vi "AlliGator Phasor Plot Multiplication Window.vi"(8 "Error In":errorcluster, 11 "Phasor Graph":refnum<vi>) -> (0 "Error Out":errorcluster, 1 "Cancelled":bool, 2 "Phasor Plot Destination Output":T1, 3 "Phasor Plot Algebra Output":T2 {"1-Exp Lifetime" min=0.0; "Delay" min=0.0})   [LabVIEW 2021, in "AlliGator Phasor Graph.lvlib"]
doc: "UI to let the user define algebraic operations to apply to Phasor Plots in the Phasor Graph."
uses:
  AlliGator Phasor Graph.lvlib
  AlliGator 2-Phasor Plot Multiplication.ctl
  Phasor/Phasor Operation.ctl
  Phasor/Phasor (g, s).ctl
  Phasor/Phasor (m, phi).ctl
  Phasor/Phasor Representation.ctl
  AlliGator Phasor Plot Destination.ctl
  Graphs/XY Graph/XY Graph Add-Ons.lvlib
  Phasor/Phasor.lvlib
panel:
  in  "Phasor Plot Destination":T1
  in  "Phasor Plot Algebra":T2 {"1-Exp Lifetime" min=0.0; "Delay" min=0.0; "Phasor Plot 2" items=["", "Phasor 1", "Phasor 2"]; "Phasor Plot 1" items=["", "Phasor 1", "Phasor 2"]}
  in  "OK":bool
  in  "Cancel":bool
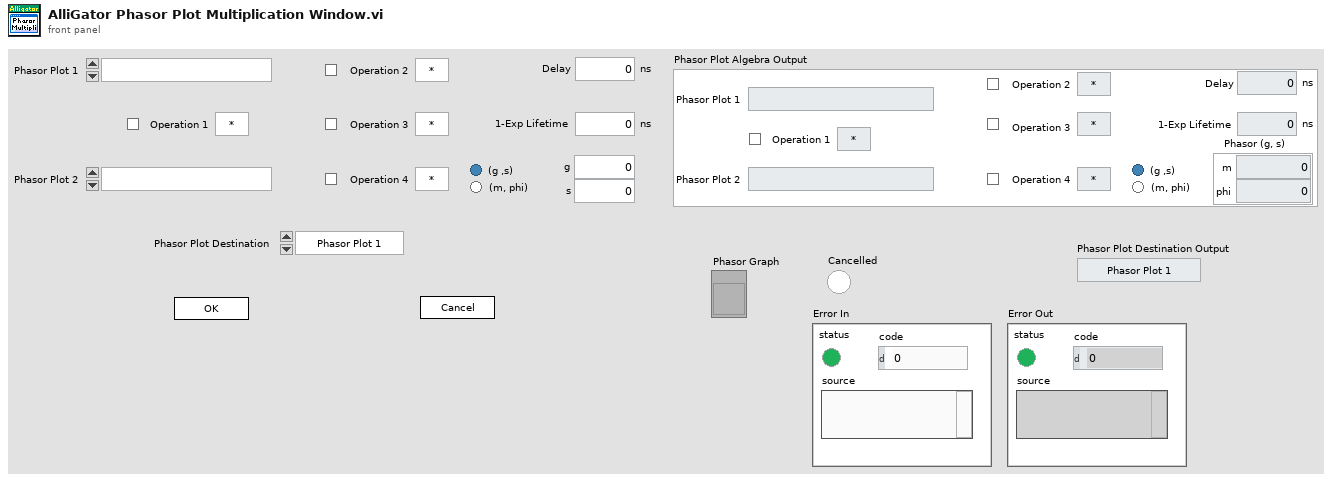
[diagram p1: front panel]
types:
  T1 = typedef "AlliGator Phasor Graph.lvlib/AlliGator Phasor Plot Destination.ctl" = enum32{"Phasor Plot 1", "Phasor Plot 2", "New Phasor Plot"}
  T2 = typedef "AlliGator Phasor Graph.lvlib/AlliGator 2-Phasor Plot Multiplication.ctl" = cluster{"Phasor Plot 1":u16, "Operation 1":T3, "Phasor Plot 2":u16, "Operation 2":T3, "Delay":dbl[unit], "Operation 3":T3, "1-Exp Lifetime":dbl[unit], "Operation 4":T3, "Phasor (g, s)":T4, "Phasor (m, phi)":T5, "Phasor Representation":T6, "Use Operation 1":bool, "Use Operation 2":bool, "Use Operation 3":bool, "Use Operation 4":bool}
  T3 = typedef "Phasor.lvlib/Phasor Operation.ctl" = enum16{"*", "/"}
  T4 = typedef "Phasor.lvlib/Phasor (g, s).ctl" = cluster{"g":dbl, "s":dbl}
  T5 = typedef "Phasor.lvlib/Phasor (m, phi).ctl" = cluster{"m":dbl, "phi":dbl}
  T6 = typedef "Phasor.lvlib/Phasor Representation.ctl" = enum32{"(g, s)", "(m, phi)"}
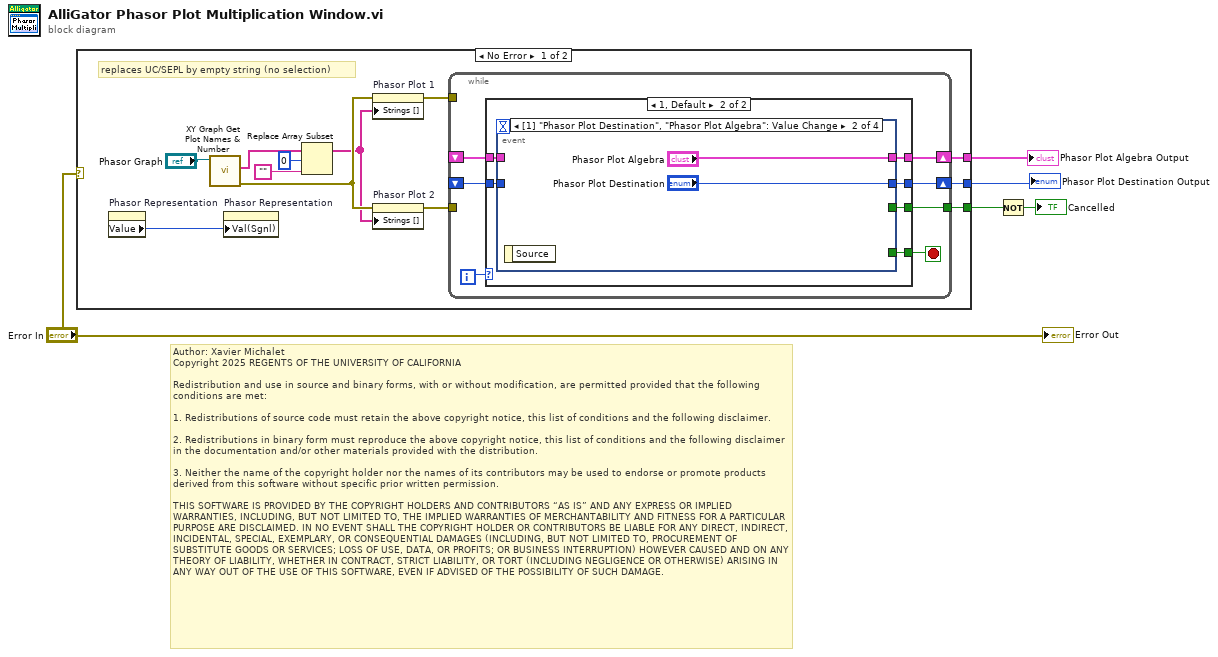
[diagram p0: block diagram]
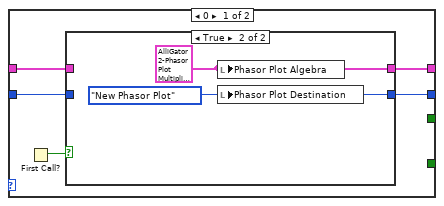
[diagram p2: hidden frame]
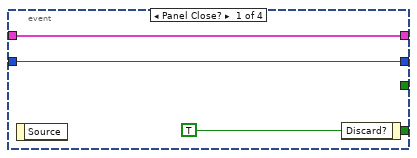
[diagram p4: hidden frame]
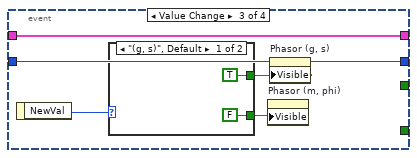
[diagram p5: hidden frame]
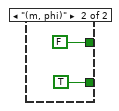
[diagram p6: hidden frame]
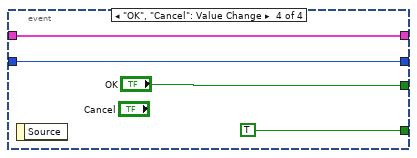
[diagram p7: hidden frame]
diagram:
  # "Author: Xavier Michalet\nCopyright 2025 REGENTS OF THE UNIVERSITY OF CALIFORNIA\n\nRedistribution and use in source and binary forms, with or without modification, are permitted provided that the following conditions are met:\n\n1. Redistributions of source code must retain the above copyright notice, this list of conditions and the following disclaimer.\n\n2. Redistributions in binary form must reproduce the above copyright notice, this list of conditions and the following disclaimer in the documentation and/or other materials provided with the distribution.\n\n3. Neither the name of the copyright holder nor the names of its contributors may be used to endorse or promote products derived from this software without specific prior written permission.\n\nTHIS SOFTWARE IS PROVIDED BY THE COPYRIGHT HOLDERS AND CONTRIBUTORS “AS IS” AND ANY EXPRESS OR IMPLIED WARRANTIES, INCLUDING, BUT NOT LIMITED TO, THE IMPLIED WARRANTIES OF MERCHANTABILITY AND FITNESS FOR A PARTICULAR PURPOSE ARE DISCLAIMED. IN NO EVENT SHALL THE COPYRIGHT HOLDER OR CONTRIBUTORS BE LIABLE FOR ANY DIRECT, INDIRECT, INCIDENTAL, SPECIAL, EXEMPLARY, OR CONSEQUENTIAL DAMAGES (INCLUDING, BUT NOT LIMITED TO, PROCUREMENT OF SUBSTITUTE GOODS OR SERVICES; LOSS OF USE, DATA, OR PROFITS; OR BUSINESS INTERRUPTION) HOWEVER CAUSED AND ON ANY THEORY OF LIABILITY, WHETHER IN CONTRACT, STRICT LIABILITY, OR TORT (INCLUDING NEGLIGENCE OR OTHERWISE) ARISING IN ANY WAY OUT OF THE USE OF THIS SOFTWARE, EVEN IF ADVISED OF THE POSSIBILITY OF SUCH DAMAGE."
  n1 = case shown="No Error" "Error In" {
    tunnel: [w17 _] -> w5
    tunnel: [w16 _] -> w3
    tunnel: [w6 _] -> w1
    frame No Error {
      # "replaces UC/SEPL by empty string (no selection)"
      n2 = property on="Phasor Representation" class="RadioBtnsControl (strict)"() -> ("Value"=w7:T6)  [unwired: 2 in, 2 out]
      n3 = call "XY Graph Get Plot Names & Number.vi"("XYGraph in"="Phasor Graph") -> ("error out"=w12:errorcluster, "Plot Names"=w11:string[])  [unwired: 5 in, 4 out]
      n4 = property on="Phasor Representation" class="RadioBtnsControl (strict)"("Val(Sgnl)"=w7) -> ()  [unwired: 2 in, 2 out]
      n5 = Replace Array Subset(array=w11, new element="", index=0) -> (w9:string[])
      n6 = property on="Phasor Plot 1" class="Ring (strict)"(error in=w12, "Strings []"=w9) -> (error out=w13:errorcluster)  [unwired: 1 in, 1 out]
      n7 = property on="Phasor Plot 2" class="Ring (strict)"(error in=w12, "Strings []"=w9) -> (error out=w14:errorcluster)  [unwired: 1 in, 1 out]
      n8 = while {
        tunnel: [w23] -> w17
        shift-right: [w22] -> w16
        shift-left: _ -> [w21]
        tunnel: w14 -> [_]
        tunnel: w13 -> [_]
        shift-right: [w20] -> w6
        shift-left: _ -> [w19]
        i -> [w18]
        stop <- w24 stop-if-true
        n9 = case shown="1, Default" w18 {
          tunnel: [_ w39] -> w24
          tunnel: [_ w38] -> w23
          tunnel: [w27 w37] -> w22
          tunnel: w21 -> [w26 w36]
          tunnel: [w28 w35] -> w20
          tunnel: w19 -> [w25 w34]
          frame 0 {
            n10 = First Call?() -> (First Call?: T/F=w29:bool)
            n11 = case shown="True" w29 {
              tunnel: [w30 w32] -> w28
              tunnel: [w31 w33] -> w27
              tunnel: w26 -> [w31 _]
              tunnel: w25 -> [w30 _]
              frame False {
              }
              frame True {
                w33 = T2 {"Phasor Plot 1"=0, "Operation 1"=enum."*", "Phasor Plot 2"=0, "Operation 2"=enum."*", "Delay"=0.0, "Operation 3"=enum."*", "1-Exp Lifetime"=0.0, "Operation 4"=enum."*", "Phasor (g, s)"={"g"=0.0, "s"=0.0}, "Phasor (m, phi)"={"m"=0.0, "phi"=0.0}, "Phasor Representation"=enum."(g, s)", "Use Operation 1"=FALSE, "Use Operation 2"=FALSE, "Use Operation 3"=FALSE, "Use Operation 4"=FALSE} ("Phasor Plot Algebra")
                w32 = AlliGator_Phasor_Plot_Destination."New Phasor Plot" ("Phasor Plot Destination")
                n12 = local write "Phasor Plot Algebra"(w33) -> ()
                n13 = local write "Phasor Plot Destination"(w32) -> ()
              }
            }
          }
          frame 1, Default {
            n14 = event shown="[1] \"Phasor Plot Destination\", \"Phasor Plot Algebra\": Value Change" {
              selector: _ -> [_ _ _ _]
              dyn-events: _ -> [_ _ _ _]
              timeout: _ -> [_ _ _ _]
              tunnel: [w42 _ _ TRUE ("Discard?")] -> w39
              tunnel: [_ _ _ "OK"] -> w38
              tunnel: [w41 "Phasor Plot Algebra" w49 w55] -> w37
              tunnel: w36 -> [w41 _ w49 w55]
              tunnel: [w40 "Phasor Plot Destination" w45 w54] -> w35
              tunnel: w34 -> [w40 _ w45 w54]
              event Panel Close? {
                w42 = TRUE ("Discard?")
                n15 = event-data() -> ()  [unwired: 1 in, 1 out]
                n16 = event-data("Discard?"=w42) -> ()  [unwired: 1 in, 1 out]
              }
              event Value Change {
                n17 = event-data() -> ()  [unwired: 1 in, 1 out]
              }
              event Value Change {
                n18 = event-data() -> ("NewVal"=w48:T6)  [unwired: 1 in]
                n19 = case shown="\"(g, s)\", Default" w48 {
                  tunnel: [TRUE ("Visible") FALSE ("Visible")] -> w47
                  tunnel: [FALSE ("Visible") TRUE ("Visible")] -> w46
                  frame "(g, s)", Default {
                  }
                  frame "(m, phi)" {
                  }
                }
                n20 = property on="Phasor (m, phi)" class="Clust (strict)"("Visible"=w46) -> ()  [unwired: 2 in, 2 out]
                n21 = property on="Phasor (g, s)" class="Clust (strict)"("Visible"=w47) -> ()  [unwired: 2 in, 2 out]
              }
              event "OK", "Cancel": Value Change {
                n22 = event-data() -> ()  [unwired: 1 in, 1 out]
              }
            }
          }
        }
      }
    }
    frame Error {
    }
  }
  "Phasor Plot Algebra Output" <- w3
  "Phasor Plot Destination Output" <- w1
  n23 = Not(x=w5) -> (.not. x?=→"Cancelled":bool)
  "Error Out" <- "Error In"
